vi "OFBS_WriteDataPaths.vi"(8 "OFBS metaparameters in":T1={"Training Data Path"=path "", "Test Data Path"=path "", "True Labels for Test Trials"=path "", "Optimization Algorithm"=enum."Genetic algorithm", "ClassifierType"=enum."Multilayer perceptron", "GA Parameters"={"Population size"=100, "Generations no."=500, "Significant digits"=4, "Crossover probabality"=0.85, "Mutation mode"=enum."one-point, fixed rate", "Use Gray code?"=FALSE, "Mutation rate"=0.05, "Min mutation rate"=0.0005, "Max mutation rate"=0.25, "Reproduction plan"=enum."Steady-state-replace-worst", "Elitism"=FALSE, "Fmax"=1}, "PSO Parameters"={"Swarm size"=50, "Generations no."=10, "Cognitive coeff a1"=2.05, "Social coeff a2"=2.05, "Min inertia weight"=0.4, "Max inertia weight "=0.9, "Fmax"=0}, "Number of Channels"=0, "Use equal number of trials?"=FALSE, "Classifier Metaparameter"=0.0, "ClassifierQualityMeasure"=enum."Accuracy"} {"Classifier Metaparameter" min=0.0 max=100.0 step=0.1 format="%#_2g"; "PSO Parameters"."Generations no." min=1; "PSO Parameters"."Swarm size" min=1; "GA Parameters"."Max mutation rate" min=0.0 max=1.0; "GA Parameters"."Min mutation rate" min=0.0 max=1.0; "GA Parameters"."Mutation rate" min=0.0 max=1.0; "GA Parameters"."Crossover probabality" min=0.0 max=1.0; "GA Parameters"."Significant digits" min=1; "GA Parameters"."Generations no." min=1; "GA Parameters"."Population size" min=1}, 11 "String Ref in":refnum<vi>) -> (0 "error out":errorcluster, 2 "String out":string, 3 "String Ref out":refnum<vi>)   [LabVIEW 2016, in "Optimal Frequency Bands Search.lvlib"]
uses:
  Optimal Frequency Bands Search.lvlib
  OFBS_metaParameters.ctl
  OFBS_AlgorithmTypes.ctl
  4. Accuracy Assessment for EEG Classification/_vlib/CU_ClassifierTypes.ctl
  GA_core/GA_tParameters.ctl
  particle_swarm_opt/PSO_tParameters.ctl
  4. Accuracy Assessment for EEG Classification/_vlib/CU_ClassifierQualityMeasure.ctl
  GA_core/GeneticAlgorithm.lvlib
  particle_swarm_opt/ParticleSwarm.lvlib
  4. Accuracy Assessment for EEG Classification/Classifier.lvlib
panel:
  # "This VI is a part of BCI Design library, http://www.ru-bci.org \nCopyright © 2020, Sotnikov Peter, All rights reserved. License: GNU GPLv3"
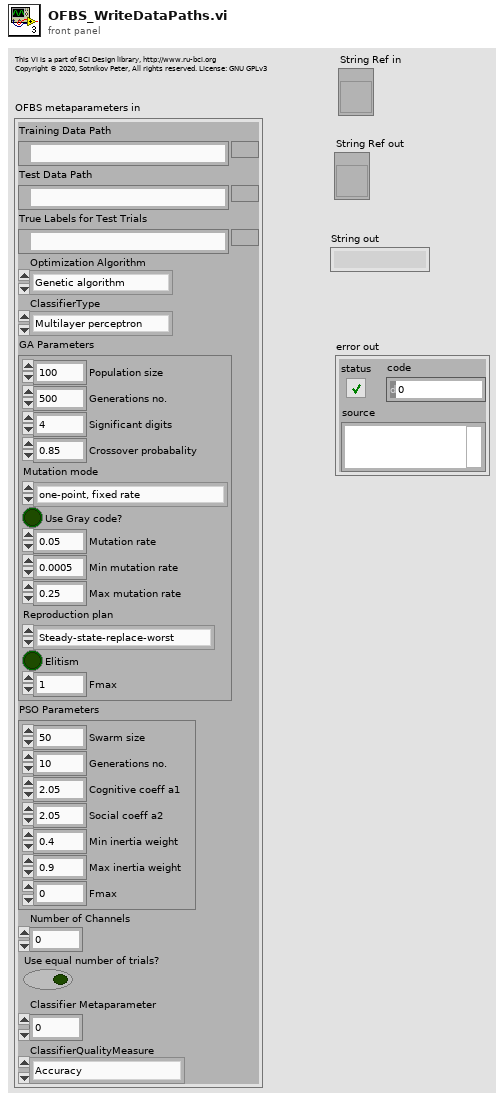
[diagram p1: front panel]
types:
  T1 = typedef "Optimal Frequency Bands Search.lvlib/OFBS_metaParameters.ctl" = cluster{"Training Data Path":path, "Test Data Path":path, "True Labels for Test Trials":path, "Optimization Algorithm":T2, "ClassifierType":T3, "GA Parameters":T4, "PSO Parameters":T5, "Number of Channels":i32, "Use equal number of trials?":bool, "Classifier Metaparameter":dbl, "ClassifierQualityMeasure":T6}
  T2 = typedef "Optimal Frequency Bands Search.lvlib/OFBS_AlgorithmTypes.ctl" = enum16{"Genetic algorithm", "Particle swarm optimization"}
  T3 = typedef "Classifier.lvlib/CU_ClassifierTypes.ctl" = enum16{"Multilayer perceptron", "k NN Classifier", "SVM Committee", "Mahalanobis distance", "SVM Classifier"}
  T4 = typedef "Optimal Frequency Bands Search.lvlib/GeneticAlgorithm.lvlib/GA_tParameters.ctl" = cluster{"Population size":i32, "Generations no.":i32, "Significant digits":i32, "Crossover probabality":dbl, "Mutation mode":enum16{"one-point, fixed rate", "one-point, fitness-adjustable rate", "one-point, distance-adjustable rate"}, "Use Gray code?":bool, "Mutation rate":dbl, "Min mutation rate":dbl, "Max mutation rate":dbl, "Reproduction plan":enum16{"Full generational replacement", "Steady-state-replace-random", "Steady-state-replace-worst"}, "Elitism":bool, "Fmax":i32}
  T5 = typedef "Optimal Frequency Bands Search.lvlib/ParticleSwarm.lvlib/PSO_tParameters.ctl" = cluster{"Swarm size":i32, "Generations no.":i32, "Cognitive coeff a1":dbl, "Social coeff a2":dbl, "Min inertia weight":dbl, "Max inertia weight ":dbl, "Fmax":i32}
  T6 = typedef "Classifier.lvlib/CU_ClassifierQualityMeasure.ctl" = enum16{"Accuracy", "Cohen's kappa"}
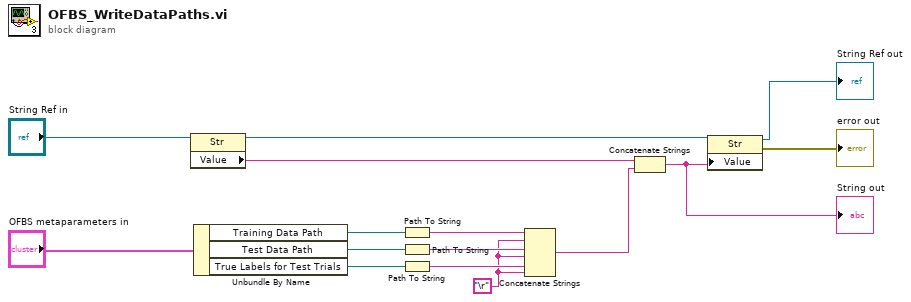
[diagram p0: block diagram]
diagram:
  w9 = "\r"
  n1 = property class="Str"(reference="String Ref in") -> (reference out=w7:refnum<vi>, "Value"=w6:string)  [unwired: 1 in, 1 out]
  n2 = Unbundle By Name("OFBS metaparameters in") -> ("Training Data Path"=w15:path, "Test Data Path"=w14:path, "True Labels for Test Trials"=w13:path)
  n3 = Path To String(path=w15) -> (string=w12:string)
  n4 = Path To String(path=w14) -> (string=w11:string)
  n5 = Path To String(path=w13) -> (string=w10:string)
  n6 = Concatenate Strings(w12, w9, w11, w9, w10, w9) -> (w5:string)
  n7 = Concatenate Strings(w6, w5) -> (w4:string)
  "String out" <- w4
  n8 = property class="Str"(reference=w7, "Value"=w4) -> (reference out=→"String Ref out":refnum<vi>, error out=→"error out":errorcluster)  [unwired: 1 in]
